vi "ElevSlowDown.vi"(8 "SlowRange":i32=16000, 9 "Target":i32, 10 "Current":i32, 11 "ElevIn":dbl) -> (3 "ElevOut":dbl)   [LabVIEW 2018]
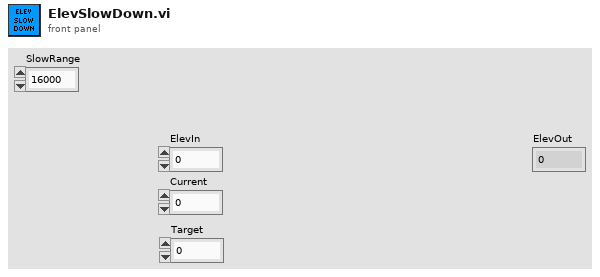
[diagram p1: front panel]
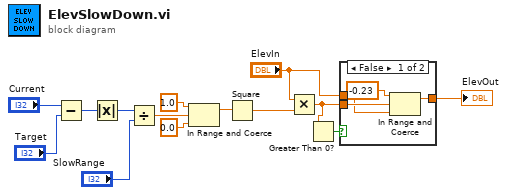
[diagram p0: block diagram]
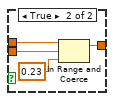
[diagram p2: hidden frame]
diagram:
  n1 = Subtract(x="Current", y="Target") -> (x-y=w12:i32)
  n2 = Absolute Value(x=w12) -> (abs(x)=w11:i32)
  n3 = Divide(x=w11, y="SlowRange") -> (x/y=w9:dbl)
  n4 = In Range and Coerce(upper limit=1.0, x=w9, lower limit=0.0) -> (coerced(x)=w2:dbl)  [unwired: 1 out]
  n5 = Square(x=w2) -> (x^2=w1:dbl)
  n6 = Multiply(x="ElevIn", y=w1) -> (x*y=w3:dbl)
  n7 = Greater Than 0?(x=w3) -> (x > 0?=w4:bool)
  n8 = case shown="False" w4 {
    tunnel: w3 -> [w17 w22]
    tunnel: [w18 w21] -> w6
    tunnel: "ElevIn" -> [w15 w20]
    frame False {
      n9 = In Range and Coerce(upper limit=-0.23 ("lower limit"), x=w17, lower limit=w15) -> (coerced(x)=w18:dbl)  [unwired: 1 out]
    }
    frame True {
      n10 = In Range and Coerce(upper limit=w20, x=w22, lower limit=0.23) -> (coerced(x)=w21:dbl)  [unwired: 1 out]
    }
  }
  "ElevOut" <- w6
